vi "rdp.vi"(5 "IN VARIANT":variant, 7 "Ip":string, 9 "Name in":string, 11 "error in (no error)":errorcluster) -> (6 "OUT VARIANT":variant, 10 "Valid data":bool, 15 "error out":errorcluster)   [LabVIEW 2015]
doc: "NON BLOCKING read operation. tuple copy is left in tuple space."
uses:
  C:/Users/Giuseppe/Downloads/LabLinda_ pakage/index_datatype.ctl
  C:/Users/Giuseppe/Downloads/LabLinda_ pakage/index_cluster.ctl
  LI_states.ctl
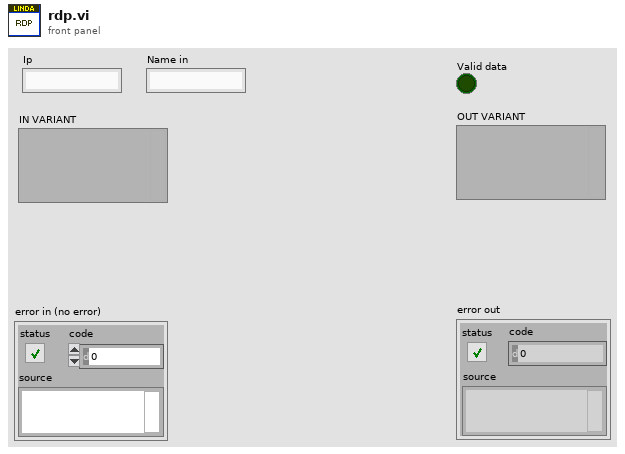
[diagram p1: front panel]
types:
  T1 = typedef "index_datatype.ctl" = T2[]
  T2 = typedef "index_cluster.ctl" = cluster{"Addr":i32[], "out react vi reference":refnum<vi>, "in react vi reference":refnum<vi>, "rd react vi reference":refnum<vi>, "Read_write_var":refnum<vi>}
  T3 = typedef "LI_states.ctl" = enum16{"Out", "In", "Rd", "Inp", "Rdp", "Init", "Cleanup", "RdAll"}
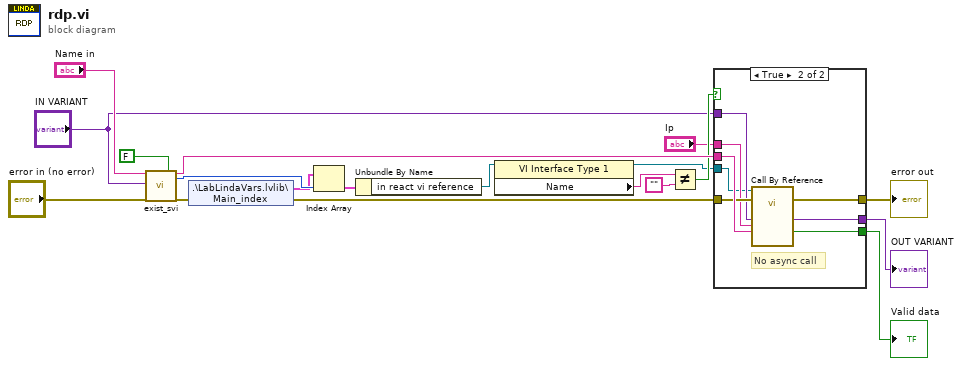
[diagram p0: block diagram]
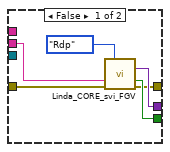
[diagram p2: hidden frame]
diagram:
  n1 = call "exist_svi.vi"("Name"="Name in", "IN VARIANT"="IN VARIANT", "error in (no error)"="error in (no error)", "Create ?"=FALSE) -> ("Name"=w14:string, "index of element"=w19:i32, "error out"=w17:errorcluster)  [unwired: 12 in, 1 out]
  n2 = shared-variable ".\\LabLindaVars.lvlib\\Main_index"(error in=w17) -> (w9:T1, error out=w6:errorcluster)
  n3 = Index Array(array=w9, index=w19) -> (element=w10:T2)
  n4 = Unbundle By Name(w10) -> ("in react vi reference"=w3:refnum<vi>)
  n5 = property class="VI Interface Type 1"(reference=w3) -> (reference out=w2:refnum<vi>, "Name"=w1:string)  [unwired: 1 in, 1 out]
  n6 = Not Equal?(x=w1, y="") -> (x != y?=w7:bool)
  n7 = case shown="True" w7 {
    tunnel: w14 -> [w23 w33]
    tunnel: w6 -> [w24 w29]
    tunnel: [w22 w31] -> w13
    tunnel: [w21 w32] -> w12
    tunnel: [w20 w30] -> w11
    tunnel: "IN VARIANT" -> [_ w28]
    tunnel: "Ip" -> [_ w27]
    tunnel: w2 -> [_ w26]
    frame False {
      n8 = call "Linda_CORE_svi_FGV.vi"("OP"=LI_states."Rdp", "Name in"=w23, "error in (no error)"=w24) -> ("OUT VARIANT"=w21:variant, "Valid Op"=w22:bool, "error out"=w20:errorcluster)  [unwired: 8 in, 2 out]
    }
    frame True {
      # "No async call"
      n9 = call-by-ref "?"(reference=w26, error in=w29, "IN VARIANT"=w28, "Ip"=w27, "Name in"=w33) -> (error out=w30:errorcluster, "OUT VARIANT"=w32:variant, "Valid data"=w31:bool)  [unwired: 10 in, 2 out]
    }
  }
  "error out" <- w11
  "Valid data" <- w13
  "OUT VARIANT" <- w12
